vi "Globals.vi"() -> ()   [LabVIEW 2015]
panel:
  out "Path":path
  out "Message window":string
  out "form type":u16
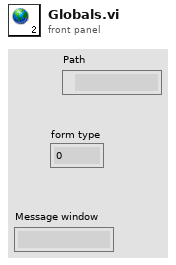
[diagram p1: front panel]
diagram:
